vi "UIRefs Flow Setpoint.vi"(8 "error in (no error)":errorcluster, 11 "FC2901 in":refnum<class "FC2901.lvclass">) -> (0 "error out":errorcluster, 3 "FC2901 out":refnum<class "FC2901.lvclass">)   [LabVIEW 2021, in "FC2901.lvclass"]
uses:
  FC2901.lvclass
  FC2901.lvclass/FC2901.ctl
  <vilib>/Utility/miscctls.llb/LVOutOfRangeActionTypeDef.ctl
  <vilib>/Utility/miscctls.llb/LVForegroundBackgroundColorsTypeDef.ctl
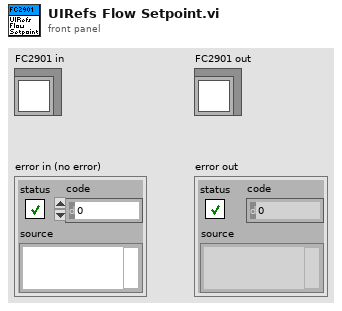
[diagram p1: front panel]
types:
  T1 = enum8{"Enabled", "Disabled", "Disabled and Grayed Out"}
  T2 = typedef "LVForegroundBackgroundColorsTypeDef.ctl" = cluster{"Foreground Color":u32, "Background Color":u32}
  T3 = typedef "LVOutOfRangeActionTypeDef.ctl" = cluster{"Out of Range Action Minimum":u8, "Out of Range Action Maximum":u8, "Out of Range Action Increment":u8}
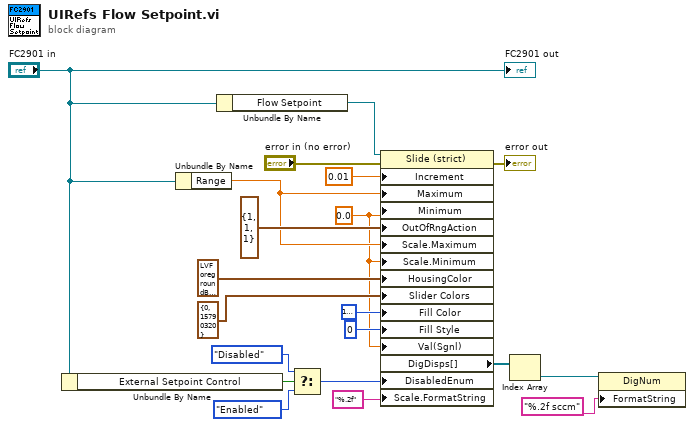
[diagram p0: block diagram]
diagram:
  w7 = 0.0 ("Data Entry Limits:Minimum")
  n1 = Unbundle By Name("FC2901 in") -> ("External Setpoint Control"=w4:bool)
  n2 = Unbundle By Name("FC2901 in") -> ("Range"=w9:dbl)
  n3 = Unbundle By Name("FC2901 in") -> ("Flow Setpoint"=w12:refnum<vi>)
  n4 = Select(t=T1."Disabled" ("Disabled"), s=w4, f=T1."Enabled") -> (s? t:f=w1:T1)
  n5 = property class="Slide (strict)"(reference=w12, error in="error in (no error)", "Increment"=0.01 ("Data Entry Limits:Increment"), "Maximum"=w9, "Minimum"=w7, "OutOfRngAction"=T3 {"Out of Range Action Minimum"=1, "Out of Range Action Maximum"=1, "Out of Range Action Increment"=1} ("Response to Value Outside Limits"), "Scale.Maximum"=w9, "Scale.Minimum"=w7, "HousingColor"=T2 {"Foreground Color"=16777216, "Background Color"=16777216} ("Housing Colors"), "Slider Colors"=T2 {"Foreground Color"=0, "Background Color"=15790320}, "Fill Color"=u32 16777216, "Fill Style"=0, "Val(Sgnl)"=w7, "DisabledEnum"=w1, "Scale.FormatString"="%.2f" ("Scale.Format String")) -> (error out=→"error out":errorcluster, "DigDisps[]"=w8:refnum<vi>[])  [unwired: 1 out]
  n6 = Index Array(array=w8) -> (element=w14:refnum<vi>)  [unwired: 1 in]
  n7 = property class="DigNum"(reference=w14, "FormatString"="%.2f sccm" ("Format String")) -> ()  [unwired: 1 in, 2 out]
  "FC2901 out" <- "FC2901 in"
